vi "WPI_DMAStart.vi"(8 "error in (no error)":errorcluster, 11 "DMARef":T1) -> (0 "error out":errorcluster, 3 "DMARef":T1)   [LabVIEW 2017]
doc: "Configures the FPGA module on the roboRIO to send all the channels you add to the DMA stream to the host computer. Also, if you pause the DMA stream using the Pause VI, this VI unpauses the stream and reinitiates the data transfer.\n\nThis software is licensed. Open the labview\\readme\\WPI Robotics Library Open Source License.txt file for more information."
uses:
  <vilib>/Rock Robotics/WPI/DMA/WPI_DMARef.ctl
  <vilib>/Rock Robotics/SystemInterfaces/DMA/FPGA_DMAEnable.ctl
  <vilib>/Rock Robotics/SystemInterfaces/DMA/FPGA_DMAWriteConfigOperation.ctl
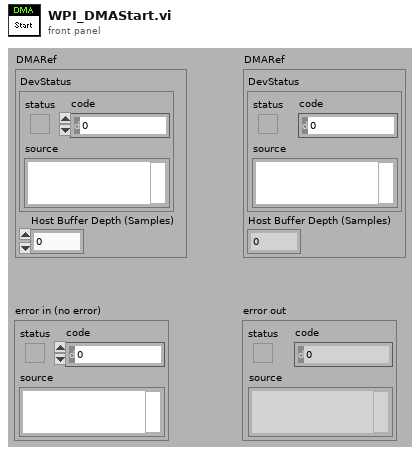
[diagram p1: front panel]
types:
  T1 = typedef "WPI_DMARef.ctl" = cluster{"DevStatus":errorcluster, "Host Buffer Depth (Samples)":u32}
  T2 = typedef "FPGA_DMAWriteConfigOperation.ctl" = enum16{"Update Pause", "Update Enable", "Update SampleClock"}
  T3 = typedef "FPGA_DMAEnable.ctl" = cluster{"AI0_Low":bool, "AI0_High":bool, "AIAveraged0_Low":bool, "AIAveraged0_High":bool, "AI1_Low":bool, "AI1_High":bool, "AIAveraged1_Low":bool, "AIAveraged1_High":bool, "Accumulator0":bool, "Accumulator1":bool, "DI":bool, "AnalogTriggers":bool, "Counters_Low":bool, "Counters_High":bool, "CounterTimers_Low":bool, "CounterTimers_High":bool, "Encoders_Low":bool, "Encoders_High":bool, "EncoderTimers_Low":bool, "EncoderTimers_High":bool}
  T4 = typedef "WPI_DMAChannelTypeEnum.ctl" = enum16{"AI (Raw)", "AI (Avg)", "Accumulator", "DI (Raw) Onboard", "DI (Filtered) Onboard", "DI (Raw) MXP", "DI (Filtered) MXP", "Analog Trigger", "Counter", "Counter (Timer)", "Encoder", "Encoder (Timer)", "Time Stamp"}
  T5 = cluster{"Channel Type":T4, "Channel Number":u8}[]
  T6 = typedef "FPGA_DMADevRef.ctl" = cluster{"DevStatus":errorcluster}
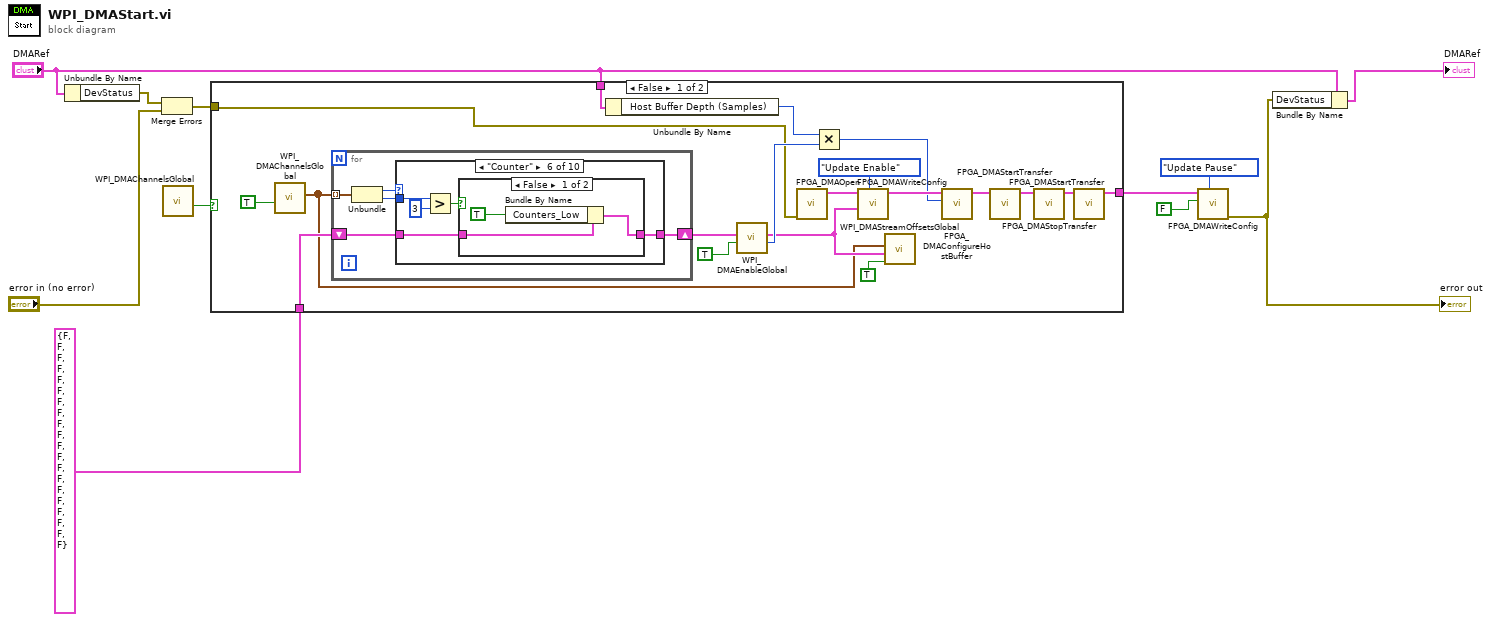
[diagram p0: block diagram]
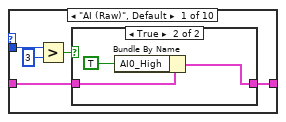
[diagram p2: hidden frame]
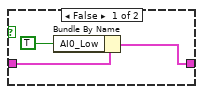
[diagram p3: hidden frame]
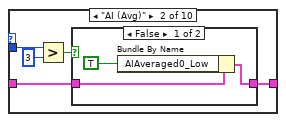
[diagram p4: hidden frame]
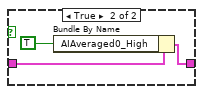
[diagram p5: hidden frame]
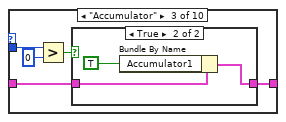
[diagram p6: hidden frame]
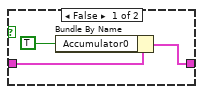
[diagram p7: hidden frame]
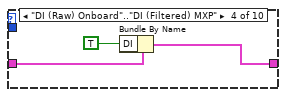
[diagram p8: hidden frame]
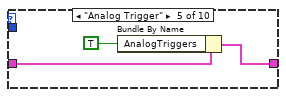
[diagram p9: hidden frame]
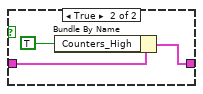
[diagram p10: hidden frame]
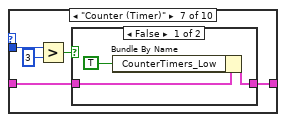
[diagram p11: hidden frame]
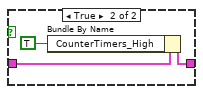
[diagram p12: hidden frame]
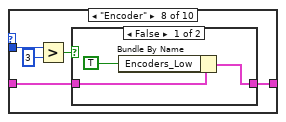
[diagram p13: hidden frame]
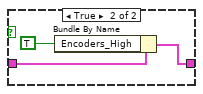
[diagram p14: hidden frame]
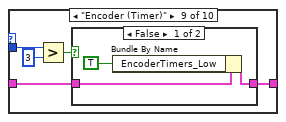
[diagram p15: hidden frame]
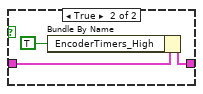
[diagram p16: hidden frame]
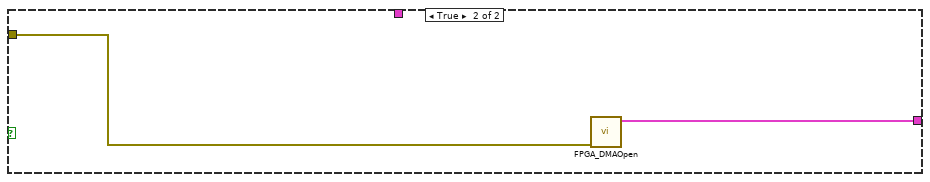
[diagram p18: hidden frame]
diagram:
  n1 = Unbundle By Name("DMARef") -> ("DevStatus"=w3:errorcluster)
  n2 = Merge Errors(w3, "error in (no error)") -> (w1:errorcluster)
  n3 = call <vilib>:"WPI_DMAChannelsGlobal.vi"() -> ("Started"=w5:bool)  [unwired: 4 in, 7 out]
  n4 = case shown="False" w5 {
    tunnel: T3 {"AI0_Low"=FALSE, "AI0_High"=FALSE, "AIAveraged0_Low"=FALSE, "AIAveraged0_High"=FALSE, "AI1_Low"=FALSE, "AI1_High"=FALSE, "AIAveraged1_Low"=FALSE, "AIAveraged1_High"=FALSE, "Accumulator0"=FALSE, "Accumulator1"=FALSE, "DI"=FALSE, "AnalogTriggers"=FALSE, "Counters_Low"=FALSE, "Counters_High"=FALSE, "CounterTimers_Low"=FALSE, "CounterTimers_High"=FALSE, "Encoders_Low"=FALSE, "Encoders_High"=FALSE, "EncoderTimers_Low"=FALSE, "EncoderTimers_High"=FALSE} ("DMA Enable") -> [w30 _]
    tunnel: "DMARef" -> [w26 _]
    tunnel: [w15 w121] -> w8
    tunnel: w1 -> [w12 w120]
    frame False {
      n5 = call <vilib>:"WPI_DMAChannelsGlobal.vi"("Start"=TRUE) -> ("Channels Out"=w17:T5)  [unwired: 3 in, 7 out]
      n6 = for {
        tunnel: w17 -> [w35] mode=indexing
        shift-right: [w31] -> w29
        shift-left: w30 -> [w32]
        n7 = Unbundle(w35) -> ("Channel Type"=w34:T4, "Channel Number"=w33:u8)
        n8 = case shown="\"Counter\"" w34 {
          tunnel: w33 -> [w40 w51 w62 _ _ w79 w90 w101 w112 _]
          tunnel: w32 -> [w38 w49 w60 w71 w74 w77 w88 w99 w110 w119]
          tunnel: [w36 w47 w58 w70 w73 w75 w86 w97 w108 w119] -> w31
          frame "AI (Raw)", Default {
            n9 = Greater?(x=w40, y=u8 3) -> (0:w37:bool)
            n10 = case shown="True" w37 {
              tunnel: w38 -> [w43 w46]
              tunnel: [w41 w44] -> w36
              frame False {
                n11 = Bundle By Name(cluster=w43, "AI0_Low"=TRUE) -> (w41:T3)
              }
              frame True {
                n12 = Bundle By Name(cluster=w46, "AI0_High"=TRUE ("AI0_Low")) -> (w44:T3)
              }
            }
          }
          frame "AI (Avg)" {
            n13 = Greater?(x=w51, y=u8 3) -> (0:w48:bool)
            n14 = case shown="False" w48 {
              tunnel: w49 -> [w54 w57]
              tunnel: [w52 w55] -> w47
              frame False {
                n15 = Bundle By Name(cluster=w54, "AIAveraged0_Low"=TRUE ("AI0_Low")) -> (w52:T3)
              }
              frame True {
                n16 = Bundle By Name(cluster=w57, "AIAveraged0_High"=TRUE ("AI0_Low")) -> (w55:T3)
              }
            }
          }
          frame "Accumulator" {
            n17 = Greater?(x=w62, y=u8 0) -> (0:w59:bool)
            n18 = case shown="True" w59 {
              tunnel: w60 -> [w65 w68]
              tunnel: [w63 w66] -> w58
              frame False {
                n19 = Bundle By Name(cluster=w65, "Accumulator0"=TRUE ("AI0_Low")) -> (w63:T3)
              }
              frame True {
                n20 = Bundle By Name(cluster=w68, "Accumulator1"=TRUE ("AI0_Low")) -> (w66:T3)
              }
            }
          }
          frame "DI (Raw) Onboard".."DI (Filtered) MXP" {
            n21 = Bundle By Name(cluster=w71, "DI"=TRUE ("AI0_Low")) -> (w70:T3)
          }
          frame "Analog Trigger" {
            n22 = Bundle By Name(cluster=w74, "AnalogTriggers"=TRUE ("AI0_Low")) -> (w73:T3)
          }
          frame "Counter" {
            n23 = Greater?(x=w79, y=u8 3) -> (0:w76:bool)
            n24 = case shown="False" w76 {
              tunnel: w77 -> [w82 w85]
              tunnel: [w80 w83] -> w75
              frame False {
                n25 = Bundle By Name(cluster=w82, "Counters_Low"=TRUE ("AI0_Low")) -> (w80:T3)
              }
              frame True {
                n26 = Bundle By Name(cluster=w85, "Counters_High"=TRUE ("AI0_Low")) -> (w83:T3)
              }
            }
          }
          frame "Counter (Timer)" {
            n27 = Greater?(x=w90, y=u8 3) -> (0:w87:bool)
            n28 = case shown="False" w87 {
              tunnel: w88 -> [w93 w96]
              tunnel: [w91 w94] -> w86
              frame False {
                n29 = Bundle By Name(cluster=w93, "CounterTimers_Low"=TRUE ("AI0_Low")) -> (w91:T3)
              }
              frame True {
                n30 = Bundle By Name(cluster=w96, "CounterTimers_High"=TRUE ("AI0_Low")) -> (w94:T3)
              }
            }
          }
          frame "Encoder" {
            n31 = Greater?(x=w101, y=u8 3) -> (0:w98:bool)
            n32 = case shown="False" w98 {
              tunnel: w99 -> [w104 w107]
              tunnel: [w102 w105] -> w97
              frame False {
                n33 = Bundle By Name(cluster=w104, "Encoders_Low"=TRUE ("AI0_Low")) -> (w102:T3)
              }
              frame True {
                n34 = Bundle By Name(cluster=w107, "Encoders_High"=TRUE ("AI0_Low")) -> (w105:T3)
              }
            }
          }
          frame "Encoder (Timer)" {
            n35 = Greater?(x=w112, y=u8 3) -> (0:w109:bool)
            n36 = case shown="False" w109 {
              tunnel: w110 -> [w115 w118]
              tunnel: [w113 w116] -> w108
              frame False {
                n37 = Bundle By Name(cluster=w115, "EncoderTimers_Low"=TRUE ("AI0_Low")) -> (w113:T3)
              }
              frame True {
                n38 = Bundle By Name(cluster=w118, "EncoderTimers_High"=TRUE ("AI0_Low")) -> (w116:T3)
              }
            }
          }
          frame "Time Stamp" {
          }
        }
      }
      n39 = Unbundle By Name(w26) -> ("Host Buffer Depth (Samples)"=w23:u32)
      n40 = call <vilib>:"WPI_DMAEnableGlobal.vi"("Set"=TRUE, "DMA Enable"=w29) -> ("WordsPerSample"=w22:u16, "DMA Enable Out"=w18:T3)  [unwired: 8 out]
      n41 = call <vilib>:"FPGA_DMAOpen.vi"("error in (no error)"=w12) -> ("DMADevRef"=w25:T6)  [unwired: 10 out]
      n42 = Multiply(x=w23, y=w22) -> (x*y=w20:u32)
      n43 = call <vilib>:"FPGA_DMAWriteConfig.vi"("Operation"=FPGA_DMAWriteConfigOperation."Update Enable", "Enable"=w18, "DMADevRef"=w25) -> ("DMADevRef"=w21:T6)  [unwired: 3 in, 5 out]
      n44 = call <vilib>:"WPI_DMAStreamOffsetsGlobal.vi"("Set"=TRUE, "Enable"=w18, "Channels"=w17) -> ()  [unwired: 9 out]
      n45 = call <vilib>:"FPGA_DMAConfigureHostBuffer.vi"("Depth"=w20, "DMADevRef In"=w21) -> ("DMADevRef Out"=w19:T6)  [unwired: 1 in, 8 out]
      n46 = call <vilib>:"FPGA_DMAStartTransfer.vi"("DMADevRef In"=w19) -> ("DMADevRef Out"=w14:T6)  [unwired: 1 in, 9 out]
      n47 = call <vilib>:"FPGA_DMAStopTransfer.vi"("DMADevRef In"=w14) -> ("DMADevRef Out"=w13:T6)  [unwired: 1 in, 9 out]
      n48 = call <vilib>:"FPGA_DMAStartTransfer.vi"("DMADevRef In"=w13) -> ("DMADevRef Out"=w15:T6)  [unwired: 1 in, 9 out]
    }
    frame True {
      n49 = call <vilib>:"FPGA_DMAOpen.vi"("error in (no error)"=w120) -> ("DMADevRef"=w121:T6)  [unwired: 10 out]
    }
  }
  n50 = call <vilib>:"FPGA_DMAWriteConfig.vi"("Operation"=FPGA_DMAWriteConfigOperation."Update Pause", "Pause"=FALSE, "DMADevRef"=w8) -> ("error out"=w11:errorcluster)  [unwired: 3 in, 5 out]
  "error out" <- w11
  n51 = Bundle By Name(cluster="DMARef", "DevStatus"=w11) -> (→"DMARef":T1)
